vi "ook_superhetero.vi"() -> ()   [LabVIEW 2009]
uses:
  <vilib>/Analysis/NI_AALBase.lvlib
panel:
  in  "雑音振幅":dbl
  out "誤り率":dbl
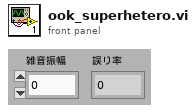
[diagram p1: front panel]
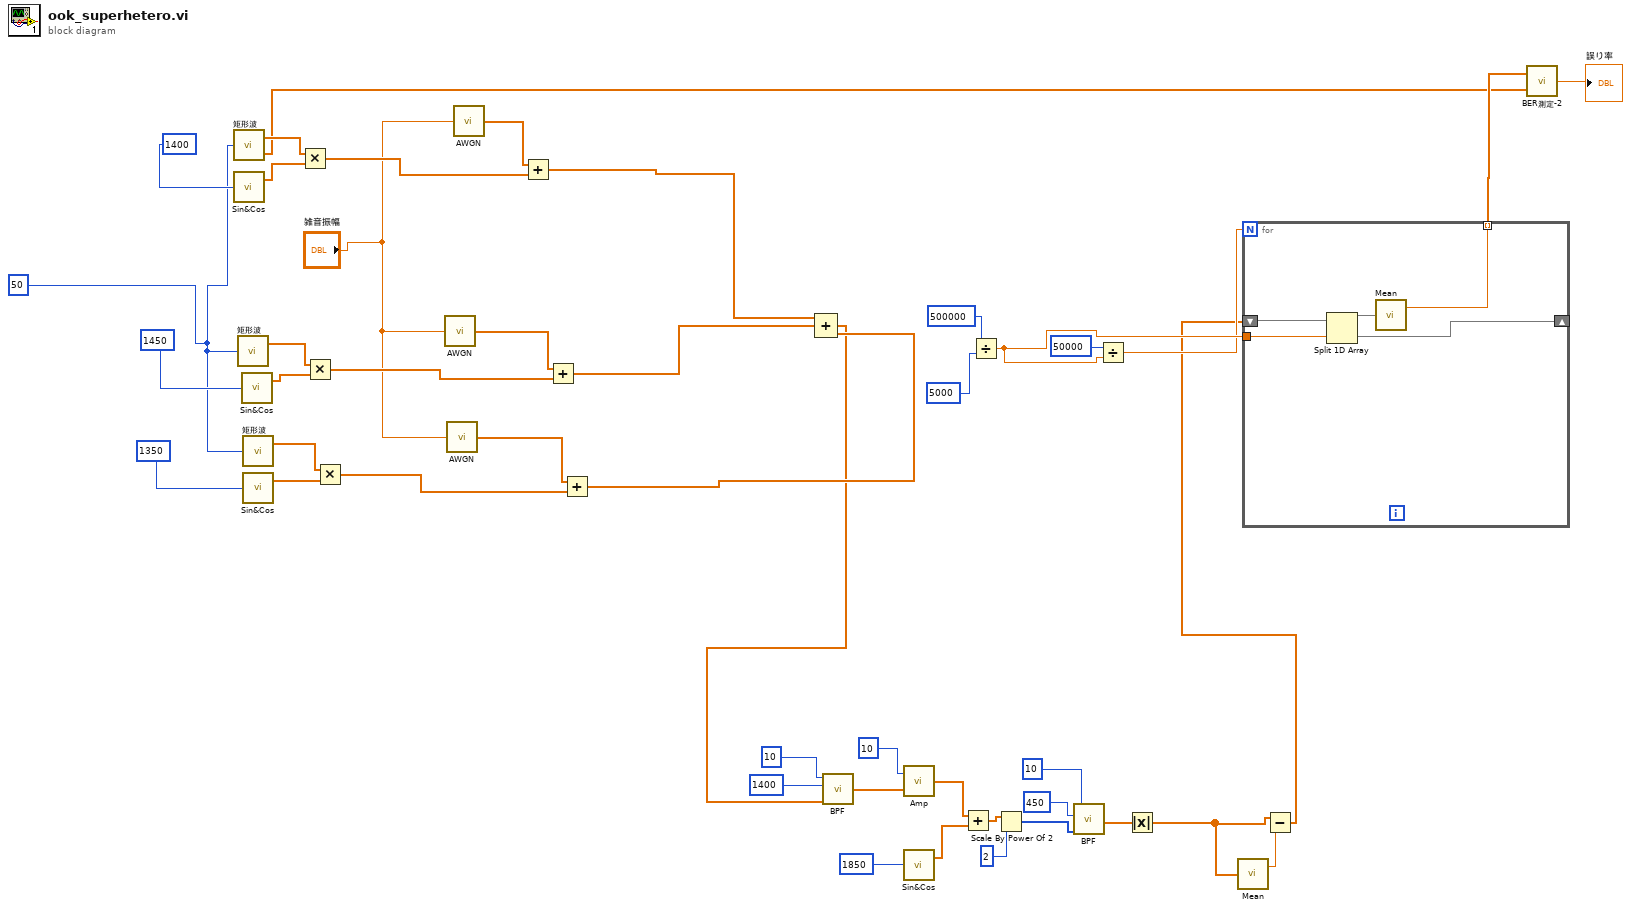
[diagram p0: block diagram]
diagram:
  w30 = 50
  n1 = call "矩形波.vi"("信号周波数 [kHz]"=w30) -> ("矩形波"=w40:dbl[], "送信データ"=w22:dbl[])
  n2 = call "Sin&Cos.vi"("周波数[kHz]"=1400) -> ("sin"=w41:dbl[])  [unwired: 1 out]
  n3 = call "矩形波.vi"("信号周波数 [kHz]"=w30) -> ("矩形波"=w43:dbl[])  [unwired: 1 out]
  n4 = call "Sin&Cos.vi"("周波数[kHz]"=1450) -> ("sin"=w42:dbl[])  [unwired: 1 out]
  n5 = call "矩形波.vi"("信号周波数 [kHz]"=w30) -> ("矩形波"=w44:dbl[])  [unwired: 1 out]
  n6 = call "Sin&Cos.vi"("周波数[kHz]"=1350) -> ("sin"=w45:dbl[])  [unwired: 1 out]
  n7 = Multiply(x=w40, y=w41) -> (x*y=w25:dbl[])
  n8 = Multiply(x=w43, y=w42) -> (x*y=w34:dbl[])
  n9 = Multiply(x=w44, y=w45) -> (x*y=w32:dbl[])
  n10 = call "AWGN.vi"("振幅値"="雑音振幅") -> ("出力"=w35:dbl[])
  n11 = call "AWGN.vi"("振幅値"="雑音振幅") -> ("出力"=w33:dbl[])
  n12 = call "AWGN.vi"("振幅値"="雑音振幅") -> ("出力"=w36:dbl[])
  n13 = Add(x=w36, y=w25) -> (x+y=w21:dbl[])
  n14 = Add(x=w35, y=w34) -> (x+y=w20:dbl[])
  n15 = Add(x=w33, y=w32) -> (x+y=w19:dbl[])
  n16 = Compound Arithmetic op=ADD(w21, w20, w19) -> (w3:dbl[])
  n17 = call "BPF.vi"("X"=w3, "中心周波数 [kHz]"=1400, "Q"=10) -> ("BPF出力"=w16:dbl[])  [unwired: 1 in]
  n18 = call "Amp.vi"("入力"=w16, "増幅率"=10) -> ("出力"=w11:dbl[])
  n19 = call "Sin&Cos.vi"("周波数[kHz]"=1850) -> ("sin"=w10:dbl[])  [unwired: 1 out]
  n20 = Add(x=w11, y=w10) -> (x+y=w13:dbl[])
  n21 = Divide(x=500000, y=5000) -> (x/y=w28:dbl)
  n22 = Scale By Power Of 2(n=w13, x=2) -> (x*2^n=w9:i32[])
  n23 = call "BPF.vi"("X"=w9, "中心周波数 [kHz]"=450, "Q"=10) -> ("BPF出力"=w5:dbl[])  [unwired: 1 in]
  n24 = Divide(x=50000, y=w28) -> (x/y=w27:dbl)
  n25 = Absolute Value(x=w5) -> (abs(x)=w1:dbl[])
  n26 = call <vilib>:"Mean.vi"("X"=w1) -> ("mean"=w4:dbl)  [unwired: 1 out]
  n27 = Subtract(x=w1, y=w4) -> (x-y=w2:dbl[])
  n28 = for {
    N: w27 -> [_]
    shift-right: [w47] -> _
    shift-left: w2 -> [w50]
    tunnel: [w48] -> w26 mode=indexing
    tunnel: w28 -> [w46]
    n29 = Split 1D Array(array=w50, index=w46) -> (first subarray=w49:dbl[], second subarray=w47:dbl[])
    n30 = call <vilib>:"Mean.vi"("X"=w49) -> ("mean"=w48:dbl)  [unwired: 1 out]
  }
  n31 = call "BER測定-2.vi"("参照データ"=w22, "入力データ"=w26) -> ("BER"=→"誤り率":dbl)
